vi "Filter Property Tree_by Type_2.vi"(10 "Show":T1, 11 "Properties for Tree":T2(array[cluster])) -> (2 "Keep?":bool[](array[boolean]), 3 "Properties for Tree":T2(array[cluster]))   [LabVIEW 2023]
panel:
  # "Same as input"
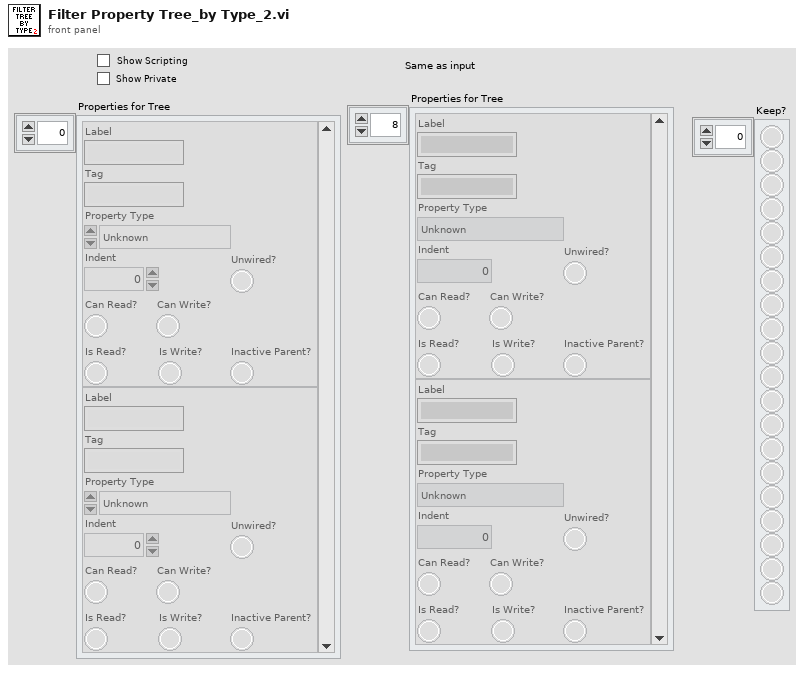
[diagram p1: front panel]
types:
  T1 = cluster{"Show Scripting":bool, "Show Private":bool}
  T2 = cluster{"Label":string, "Tag":string, "Property Type":enum16{"Unknown", "Base", "Scripting", "Private", "Deprecated", "None", "Divider"}, "Indent":u16, "Can Read?":bool, "Can Write?":bool, "Is Read?":bool, "Is Write?":bool, "Inactive Parent?":bool, "Unwired?":bool}[]
  T3 = enum16{"Unknown", "Base", "Scripting", "Private", "Deprecated", "None", "Divider"}
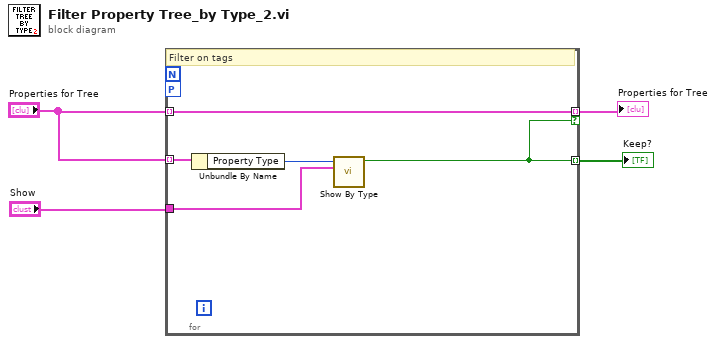
[diagram p0: block diagram]
diagram:
  n1 = for {
    tunnel: "Show" -> [w9]
    workers-P: _ -> [_]
    tunnel: "Properties for Tree" -> [w8] mode=indexing
    tunnel: [w5] -> w4 mode=indexing
    tunnel: "Properties for Tree" -> [w6] mode=indexing
    tunnel: [w6] -> w1 mode=indexing if=w5
    # "Filter on tags"
    n2 = Unbundle By Name(w8) -> ("Property Type"=w7:T3)
    n3 = call "Show By Type.vi"("Show"=w9, "Item's Property Type"=w7) -> ("Show"=w5:bool)  [unwired: 9 in]
  }
  "Properties for Tree" <- w1
  "Keep?" <- w4
